vi "LVtoInfluxDBTS.vi"(1 "LV Timestamp":timestamp) -> (0 "InfluxDB ns Timestamp":string)   [LabVIEW 2013, in "ovenCtrl.lvlib"]
uses:
  ovenCtrl.lvlib
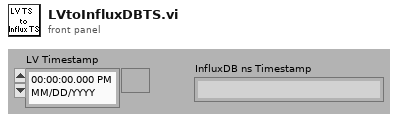
[diagram p1: front panel]
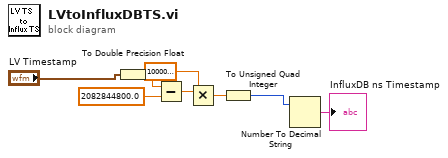
[diagram p0: block diagram]
diagram:
  n1 = To Double Precision Float(number="LV Timestamp") -> (double precision float=w7:dbl)
  n2 = Subtract(x=w7, y=2082844800.0) -> (x-y=w5:dbl)
  n3 = Multiply(x=w5, y=1000000000.0) -> (x*y=w3:dbl)
  n4 = To Unsigned Quad Integer(1:w3) -> (0:w2:u64)
  n5 = Number To Decimal String(number=w2) -> (decimal integer string=→"InfluxDB ns Timestamp":string)  [unwired: 1 in]
